vi "Line Pokayoke.vi"(8 "error in (no error)":errorcluster, 11 "Ref In":T6={"MS SQL Connection"=refnum, "UDL File"=path "", "Time"="", "DCODE"="", "WIP+1"=0, "MC No?"=0, "POKAYOKE?"=FALSE, "Expected Result"="", "Result [Status]"="", "Clock"=0.0, "RFID"="", "WIP Queue"=refnum, "TS Parameter"={"ProfitCenterCode"="", "LineCode"="", "WorkOrderNumber"="", "Model"="", "Model_with_Prefix"="", "VendorCode"="", "SetParameterDateCode"="", "PokaYoke"=0, "Target"=1, "Live_DateCode"="", "CustomerPartNumber"="", "Hand"="", "sBarcode"=FALSE, "FCA"=0, "Ent_Stamp"=timestamp(0 s since 1904-01-01), "STS_CD"=0.0}, "Data_Queue"=[], "RFID Serial No."=""} {"TS Parameter"."FCA" format="%01d"; "TS Parameter"."Target" min=1 max=100000; "TS Parameter"."PokaYoke" min=0 max=1}) -> (0 "error out":errorcluster)   [LabVIEW 2020]
uses:
  Controls/TD SQL.ctl
  <vilib>/addons/database/Connection.llb/Conn ObjectReference.ctl
  Controls/WIP_State.ctl
  Controls/TS_Parameter.ctl
  Controls/Line_PKYK.ctl
  Controls/PARA_CONTROL_STR.ctl
  Controls/PKYK_MCODE.ctl
  Controls/PKYK_DATE.ctl
  Controls/PKYK_Result.ctl
  <vilib>/Utility/miscctls.llb/LVPointTypeDef.ctl
  <vilib>/addons/database/Connection.llb/Conn Execute.vi
  <vilib>/addons/database/Recordset.llb/Rec Fetch Recordset Data (R).vi
  <vilib>/addons/database/NI_Database_API.lvlib
panel:
  in  "Hide":bool
  in  "OperationCode":T1 caption="Machine Code" items=["OP00", "OP10A", "OP10B", "OP20A", "OP20B", "OP30A", "OP30B", "OP30C", "OP40A", "OP40B", "OP50A", "OP50B", "OP60", "OP70", "OP80"]
  in  "MachineCode":T1 caption="Machine Code" items=["MCIG", "MCPC", "MCSA", "MCCA", "MCAC", "MCLA", "MCCM", "MCSC", "MCPA", "MCLP", "MCHP", "MCBC", "MCFA", "MCSR", "MCFV"]
  in  "PokaYokeNumber":string caption="PokaYoke Number"
  in  "Barcode":string
  in  "Part Number":string(combo)
  in  "PokaYoke Number":u16(ring) caption="PokaYokeNumber" items=["<New PokaYoke>", "00001", "00002", "00003", "00004", "00005", "00006", "00007", "00008", "00009", "00010", "00011", "00012", "00013", "00014", "00015", "00016"]
  in  "ExpiryDate":timestamp caption="Expiry Date" format="%<%d-%m-%Y>T"
  in  "Expected Result":T2
  in  "Description":string
  in  "Active Status":bool caption="IsActive"
  out "Date:":string
  out "Time:":string
  in  "Final Table":i32(listbox)
  in  "Refresh":bool
  in  "Print":bool
  in  "Exit":bool
  in  "Del":bool
  in  "change":bool
  in  "add":bool
  in  "PokaYoke Parameter":T3 {"MachineCode" items=["MCIG", "MCPC", "MCSA", "MCCA", "MCAC", "MCLA", "MCCM", "MCSC", "MCPA", "MCLP", "MCHP", "MCBC", "MCFA", "MCSR", "MCFV"]; "ExpiryDate" format="%<%I:%M:%S%3u %p\n%d-%m-%Y>T"; "EntDt" format="%<%I:%M:%S%3u %p\n%d-%m-%Y>T"; "UpdDt" format="%<%I:%M:%S%3u %p\n%d-%m-%Y>T"}
  # "Line Pokayoke"
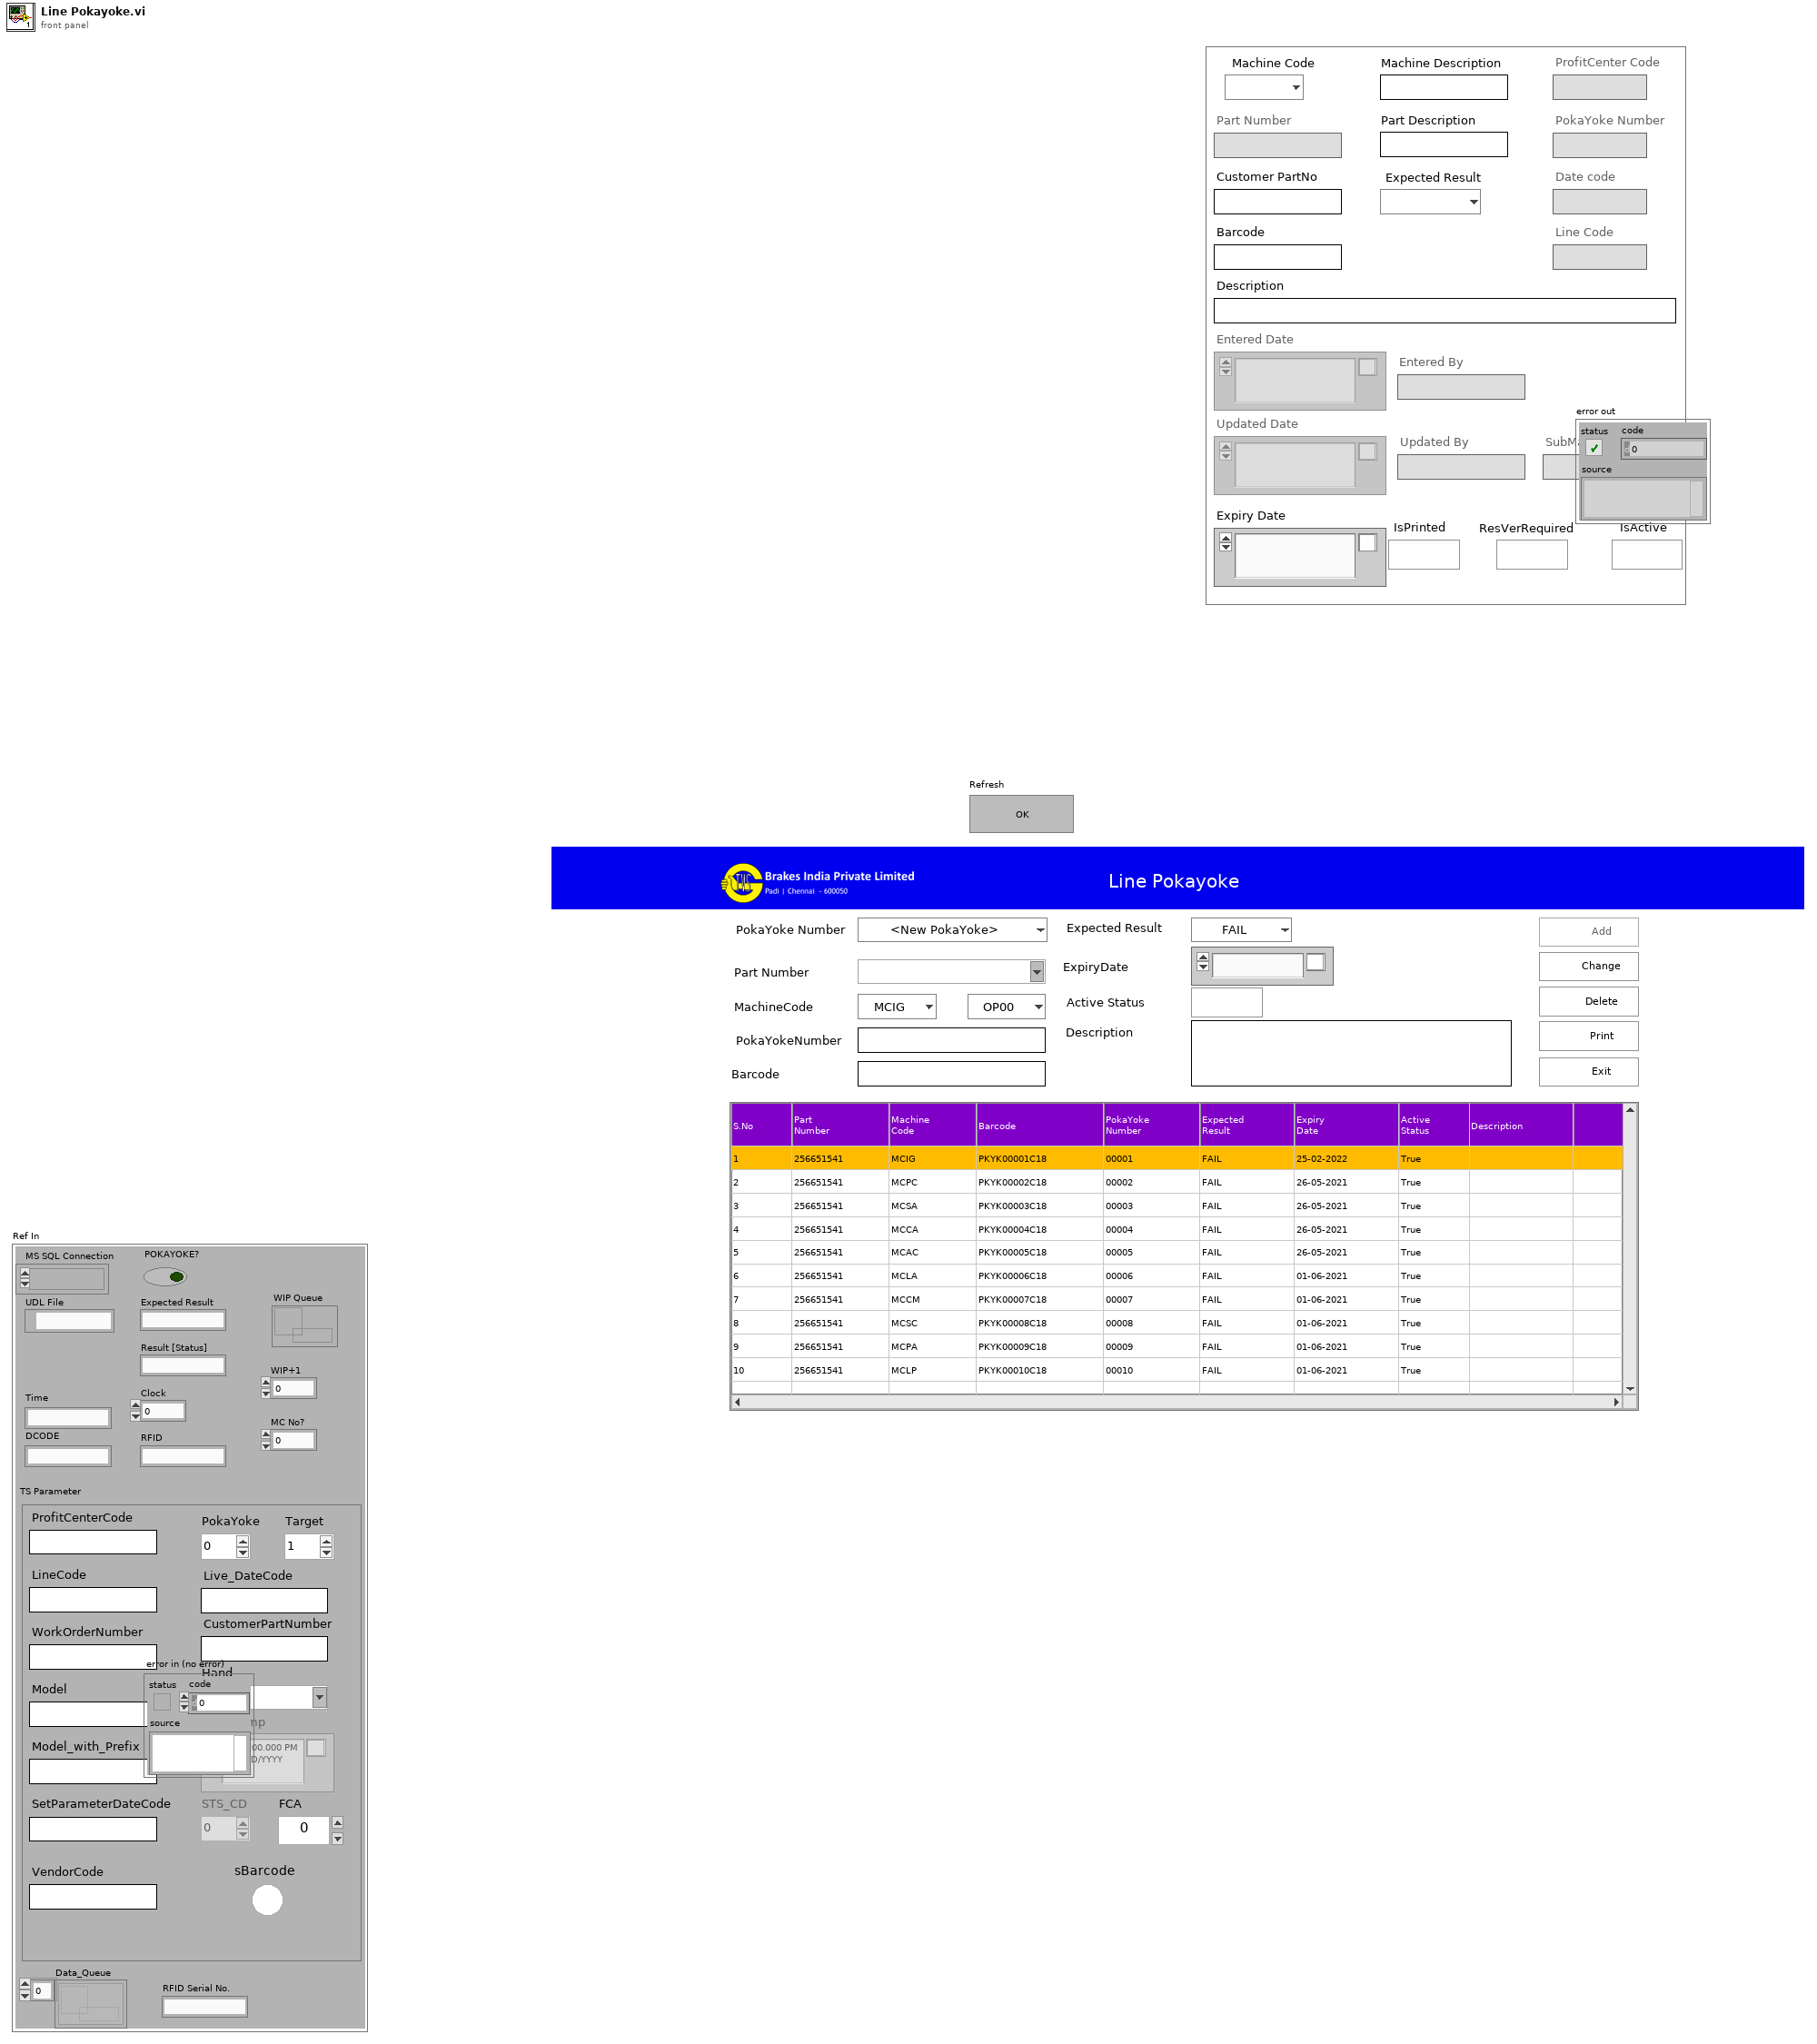
[diagram p1: front panel]
types:
  T1 = typedef "PKYK_MCODE.ctl" = u16
  T2 = typedef "PKYK_Result.ctl" = enum16{"FAIL", "PASS"}
  T3 = typedef "Line_PKYK.ctl" = cluster{"ProfitCenterCode":string, "LineCode":string, "Datecode":string, "PartNumber":T4, "PartDescription":T4, "CustPartNo":T4, "MachineCode":T1, "MachineDescription":T4, "PokaYokeNumber":string, "Description":string, "ExpiryDate":T5, "Barcode":T4, "IsPrinted":bool, "IsActive":bool, "EntBy":T4, "EntDt":T5, "UpdBy":T4, "UpdDt":T5, "ExpResult":T2, "ResVerRequired":bool, "SubMachineCode":T4}
  T4 = typedef "PARA_CONTROL_STR.ctl" = string
  T5 = typedef "PKYK_DATE.ctl" = timestamp
  T6 = typedef "TD SQL.ctl" = cluster{"MS SQL Connection":T7, "UDL File":path, "Time":string, "DCODE":string, "WIP+1":i64, "MC No?":i32, "POKAYOKE?":bool, "Expected Result":string, "Result [Status]":string, "Clock":dbl, "RFID":string, "WIP Queue":refnum<queue>, "TS Parameter":T8, "Data_Queue":refnum<queue>[], "RFID Serial No.":string}
  T7 = typedef "NI_Database_API.lvlib/Conn ObjectReference.ctl" = refnum<k1>
  T8 = typedef "TS_Parameter.ctl" = cluster{"ProfitCenterCode":string, "LineCode":string, "WorkOrderNumber":string, "Model":string, "Model_with_Prefix":string, "VendorCode":string, "SetParameterDateCode":string, "PokaYoke":i32, "Target":i32, "Live_DateCode":string, "CustomerPartNumber":string, "Hand":string, "sBarcode":bool, "FCA":i32, "Ent_Stamp":timestamp, "STS_CD":dbl}
  T9 = typedef "LVPointTypeDef.ctl" = cluster{"Horizontal":i16, "Vertical":i16}
  T10 = enum8{"Enabled", "Disabled", "Disabled and Grayed Out"}
  T11 = typedef "LVDateTimeRec.ctl" = cluster{"fractional second":dbl, "second":i32, "minute":i32, "hour":i32, "day of month":i32, "month":i32, "year":i32, "day of week":i32, "day of year":i32, "DST":i32}
  T12 = cluster{"s.nO":i32, "PartNumber":string, "MachineCode":string, "Barcode":string, "PokaYokeNumber":string, "ExpResult":string, "ExpiryDate":timestamp, "IsActive":bool, "Description":string}
  T13 = typedef "NI_Database_API.lvlib/Rec ObjectReference.ctl" = refnum<k1>
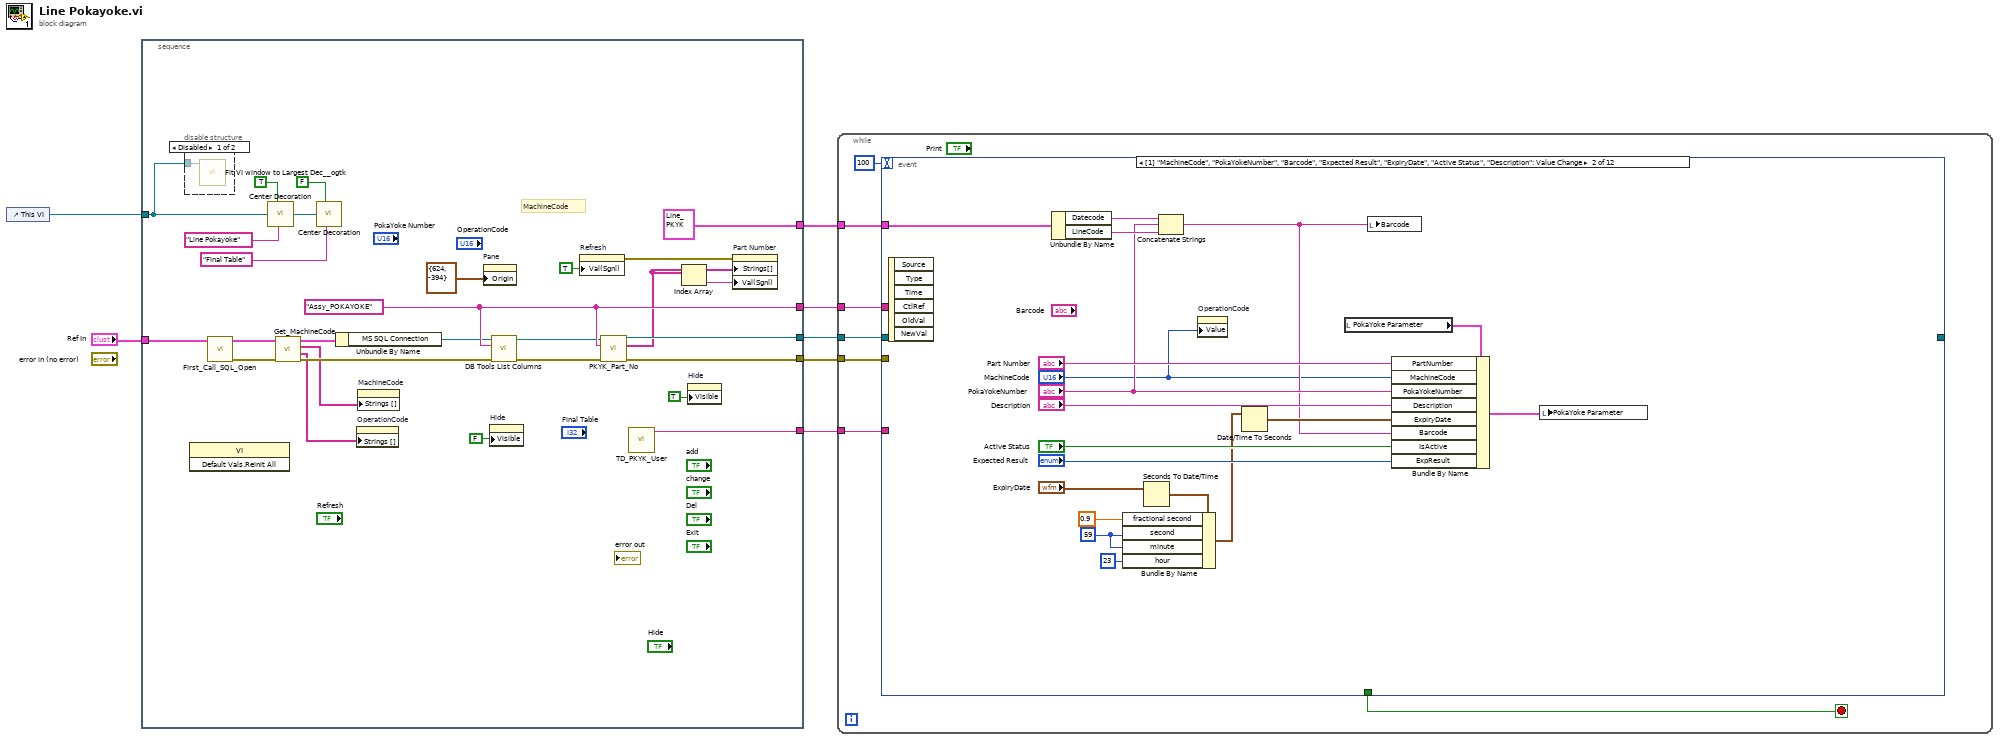
[diagram p0: block diagram]
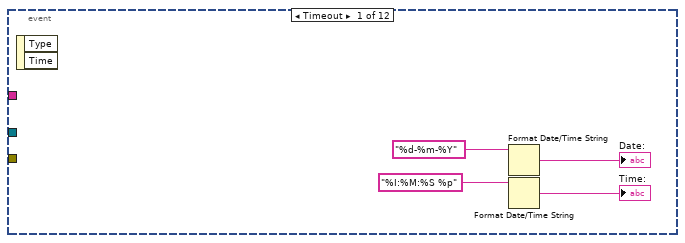
[diagram p2: hidden frame]
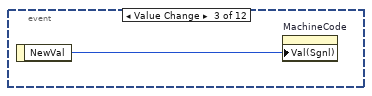
[diagram p3: hidden frame]
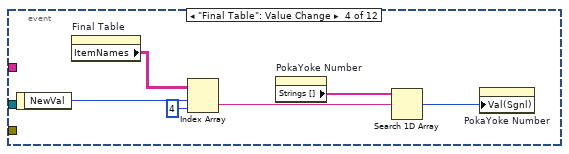
[diagram p4: hidden frame]
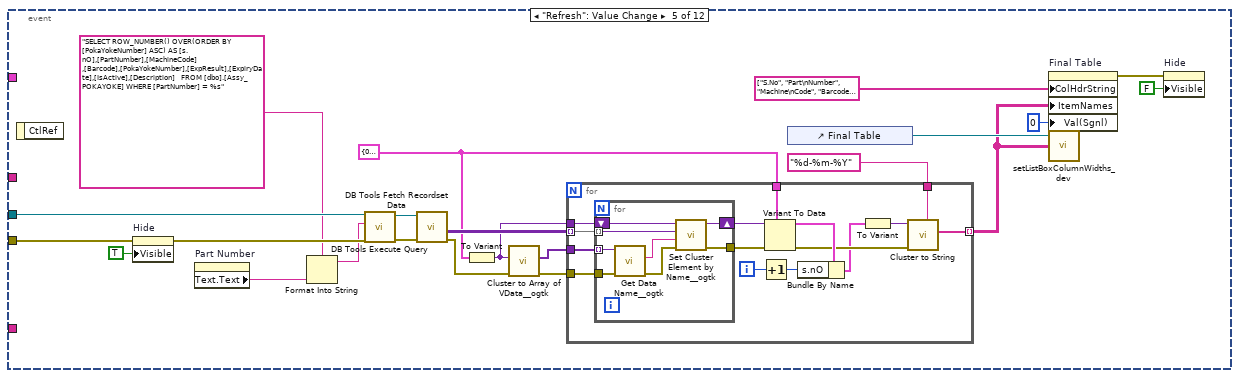
[diagram p5: hidden frame]
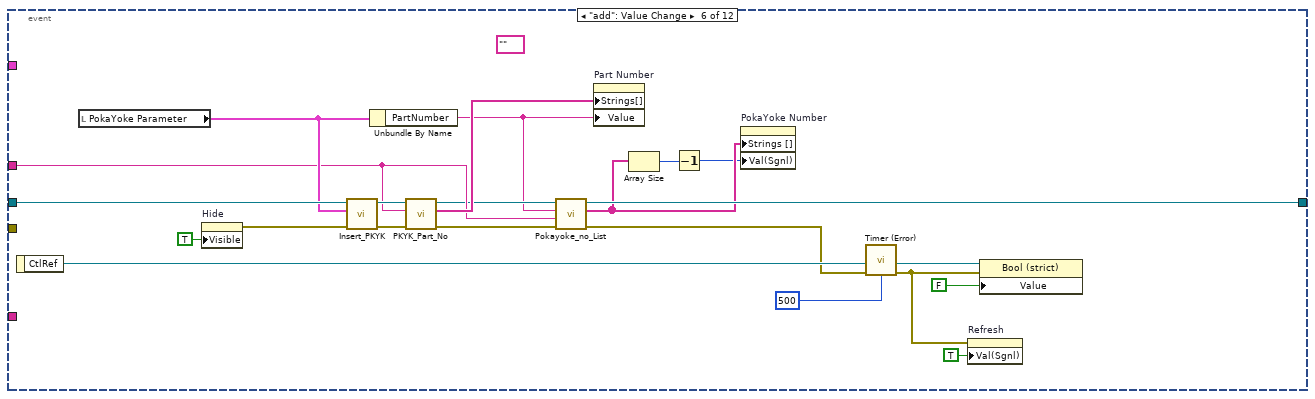
[diagram p6: hidden frame]
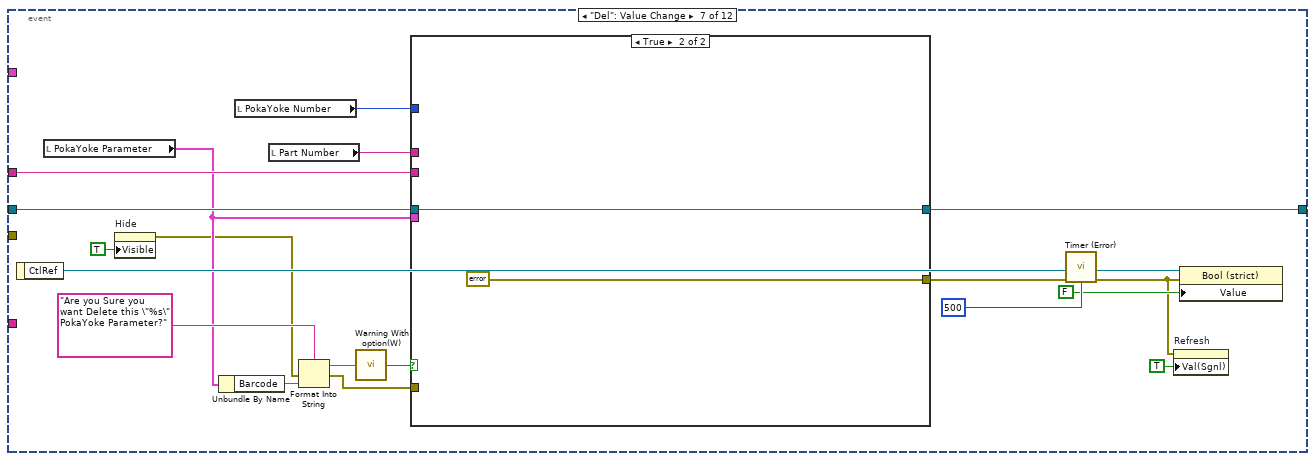
[diagram p7: hidden frame]
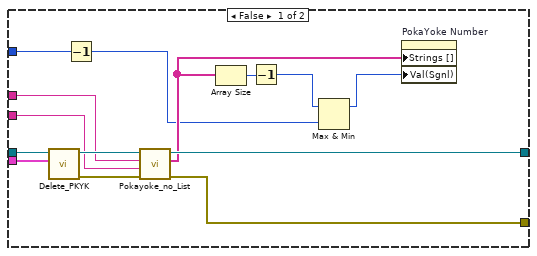
[diagram p8: hidden frame]
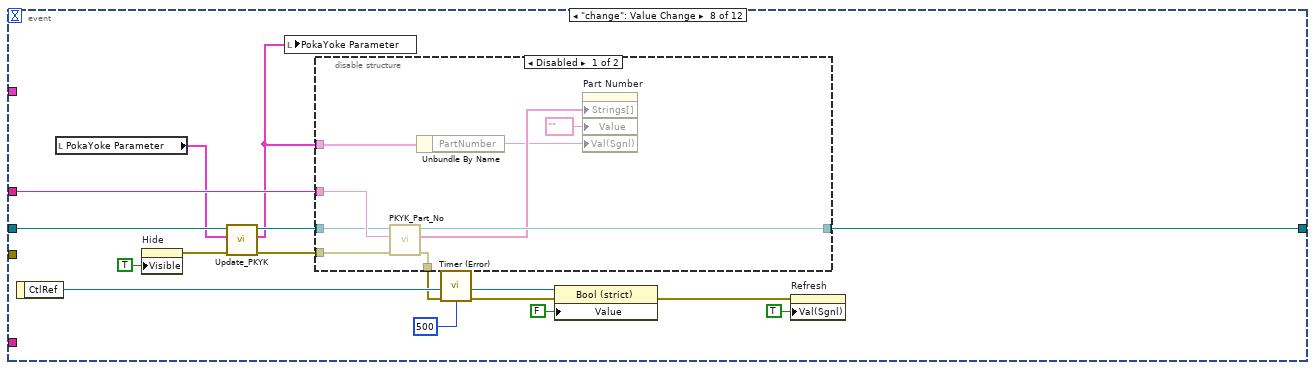
[diagram p9: hidden frame]
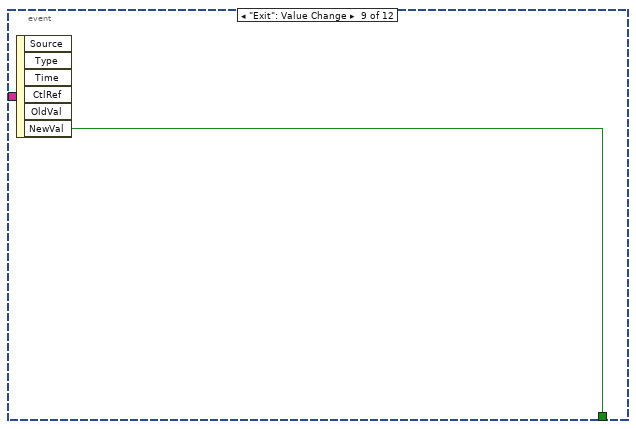
[diagram p11: hidden frame]
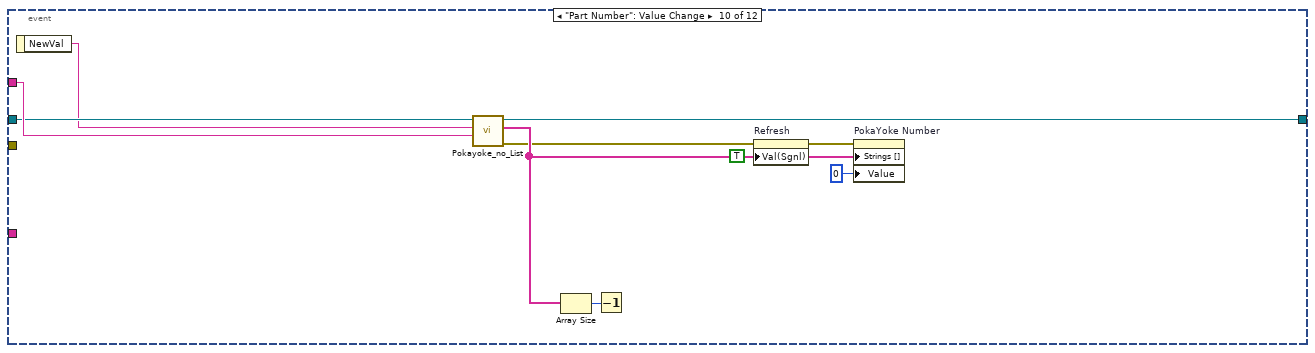
[diagram p12: hidden frame]
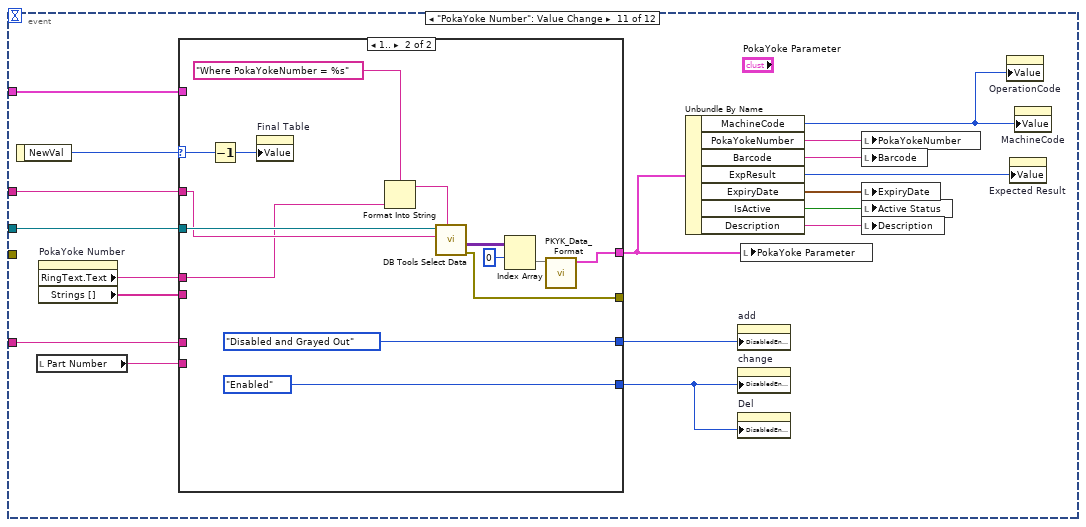
[diagram p13: hidden frame]
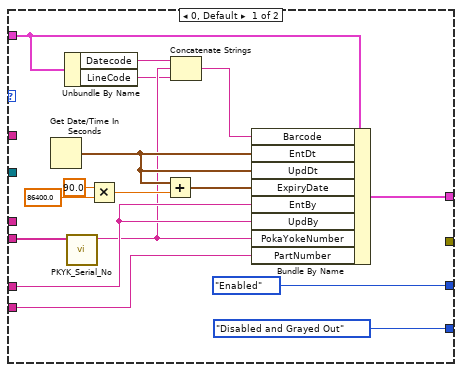
[diagram p14: hidden frame]
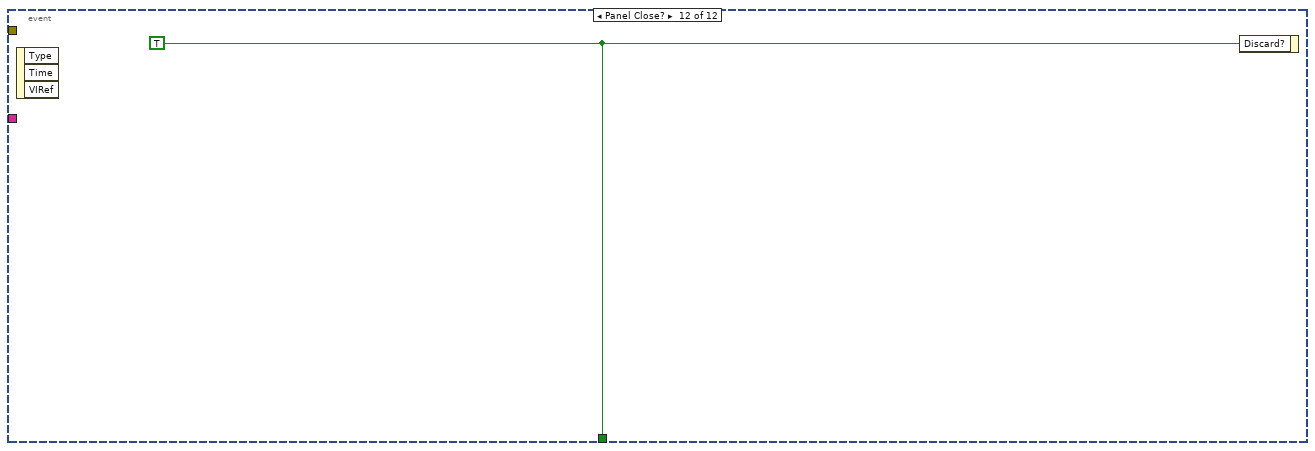
[diagram p15: hidden frame]
diagram:
  n1 = control-ref of="This VI"() -> (w1:refnum<vi>)
  n2 = stacked-sequence {
    tunnel: "Ref In" -> [w16]
    tunnel: [w34] -> w6
    tunnel: [w33] -> w5
    tunnel: [w32] -> w4
    tunnel: [T3 {"ProfitCenterCode"="0064", "LineCode"="C10", "Datecode"="PKYK", "PartNumber"="", "PartDescription"="", "CustPartNo"="", "MachineCode"=0, "MachineDescription"="", "PokaYokeNumber"="00008", "Description"="", "ExpiryDate"=timestamp(0 s since 1904-01-01), "Barcode"="PKYK00008C10", "IsPrinted"=TRUE, "IsActive"=TRUE, "EntBy"="ADMIN", "EntDt"=timestamp(0 s since 1904-01-01), "UpdBy"="ADMIN", "UpdDt"=timestamp(0 s since 1904-01-01), "ExpResult"=enum."FAIL", "ResVerRequired"=TRUE, "SubMachineCode"=""} ("Machine Code")] -> w3
    tunnel: [w26] -> w2
    tunnel: w1 -> [w13]
    frame #0 {
      w33 = "Assy_POKAYOKE" ("table")
      # "MachineCode"
      n3 = disable-structure shown="Disabled" {
        disable-tunnel: w13 -> [w36 _]
        frame Disabled {
          n4 = call <userlib>:"Fit VI window to Largest Dec__ogtk.vi"("VI Ref (calling VI)"=w36) -> ()  [unwired: 5 in, 2 out]
        }
        frame Enabled {
        }
      }
      n5 = invoke class="VI" method="Default Vals.Reinit All"() -> ()  [unwired: 3 in, 3 out]
      n6 = call "First_Call_SQL_Open.vi"("Ref In"=w16) -> ("error out"=w14:errorcluster, "Ref Out"=w15:T6)  [unwired: 9 in]
      n7 = call "Center Decoration.vi"("Decoration?"=TRUE, "VI in"=w13, "Object Name"="Line Pokayoke") -> ("VI out"=w10:refnum<vi>)  [unwired: 6 in]
      n8 = call "Get_MachineCode.vi"("error in (no error)"=w14, "Ref In"=w15) -> ("error out"=w19:errorcluster, "OperationCode"=w17:string[], "Machine Codes"=w18:string[], "Ref Out"=w20:T6)  [unwired: 6 in]
      n9 = call "Center Decoration.vi"("Decoration?"=FALSE, "VI in"=w10, "Object Name"="Final Table") -> ()  [unwired: 6 in, 1 out]
      n10 = Unbundle By Name(w20) -> ("MS SQL Connection"=w28:T7)
      n11 = property on="OperationCode" class="Ring (strict)"("Strings []"=w17) -> ()  [unwired: 2 in, 2 out]
      n12 = property on="MachineCode" class="Ring (strict)"("Strings []"=w18) -> ()  [unwired: 2 in, 2 out]
      n13 = property on="Pane" class="Pane"("Origin"=T9 {"Horizontal"=624, "Vertical"=-394}) -> ()  [unwired: 2 in, 2 out]
      n14 = property on="Hide" class="Bool"("Visible"=FALSE) -> ()  [unwired: 2 in, 2 out]
      n15 = call <vilib>:"DB Tools List Columns.vi"("error in (no error)"=w19, "table"=w33, "connection reference"=w28) -> ("error out"=w35:errorcluster, "connection reference out"=w27:T7)  [unwired: 1 in, 2 out]
      n16 = property on="Refresh" class="Bool (strict)"("Val(Sgnl)"=TRUE ("Value (Signaling)")) -> (error out=w24:errorcluster)  [unwired: 2 in, 1 out]
      n17 = call "PKYK_Part_No.vi"("error in (no error)"=w35, "table"=w33, "Refnum in"=w27) -> ("error out"=w26:errorcluster, "PKYK Part Number"=w31:string[], "Refnum out"=w34:T7)  [unwired: 6 in]
      n18 = call "TD_PKYK_User.vi"() -> ("User"=w32:string)  [unwired: 11 in]
      n19 = Index Array(array=w31) -> (element=w30:string)  [unwired: 1 in]
      n20 = property on="Hide" class="Bool"("Visible"=TRUE) -> ()  [unwired: 2 in, 2 out]
      n21 = property on="Part Number" class="CmbBox"(error in=w24, "Strings[]"=w31, "Val(Sgnl)"=w30) -> ()  [unwired: 1 in, 2 out]
    }
  }
  n22 = while {
    tunnel: w6 -> [w42]
    tunnel: w5 -> [w41]
    tunnel: w4 -> [w40]
    tunnel: w3 -> [w39]
    tunnel: w2 -> [w38]
    stop <- w43 stop-if-true
    n23 = event shown="[1] \"MachineCode\", \"PokaYokeNumber\", \"Barcode\", \"Expected Result\", \"ExpiryDate\", \"Active Status\", \"Description\": Value Change" {
      selector: _ -> [_ _ _ _ _ _ _ _ _ _ _ _]
      dyn-events: _ -> [_ _ _ _ _ _ _ _ _ _ _ _]
      timeout: 100 -> [_ _ _ _ _ _ _ _ _ _ _ _]
      tunnel: [_ _ _ _ _ _ _ _ w201 _ _ w260] -> w43
      tunnel: w42 -> [_ _ _ _ w95 w139 w158 w190 _ w210 w228 _]
      tunnel: w41 -> [_ _ _ _ _ w127 w155 w185 _ w211 w227 _]
      tunnel: w40 -> [_ _ _ _ _ _ _ _ _ _ w225 _]
      tunnel: w39 -> [_ w51 _ _ _ _ _ _ _ _ w224 _]
      tunnel: [_ _ _ _ _ w124 w154 w182 _ w206 _ _] -> _
      tunnel: w38 -> [_ _ _ _ w85 _ _ _ _ _ _ _]
      event Timeout {
        n24 = event-data() -> ()  [unwired: 1 in, 2 out]
        n25 = Format Date/Time String(time format string (%c)="%d-%m-%Y") -> (date/time string=→"Date:":string)  [unwired: 2 in]
        n26 = Format Date/Time String(time format string (%c)="%I:%M:%S %p") -> (date/time string=→"Time:":string)  [unwired: 2 in]
      }
      event "PokaYokeNumber", "Barcode", "ExpiryDate", "Active Status", "Description": Value Change {
        w55 = 59 ("second")
        n27 = event-data() -> ()  [unwired: 1 in, 6 out]
        n28 = Unbundle By Name(w51) -> ("Datecode"=w53:string, "LineCode"=w52:string)
        n29 = Seconds To Date/Time(time stamp (now)="ExpiryDate") -> (date time rec=w59:T11)  [unwired: 1 in]
        n30 = Bundle By Name(cluster=w59, "fractional second"=0.9, "second"=w55, "minute"=w55, "hour"=23) -> (w57:T11)
        n31 = Concatenate Strings(w53, "PokaYokeNumber", w52) -> (w49:string)
        n32 = property on="OperationCode" class="Ring (strict)"("Value"="MachineCode") -> ()  [unwired: 2 in, 2 out]
        n33 = Date/Time To Seconds(2:w57) -> (0:w58:timestamp)  [unwired: 1 in]
        n34 = local read "PokaYoke Parameter"() -> (w66:T3)
        n35 = local write "Barcode"(w49) -> ()
        n36 = Bundle By Name(cluster=w66, "PartNumber"="Part Number", "MachineCode"="MachineCode", "PokaYokeNumber"="PokaYokeNumber", "Description"="Description", "ExpiryDate"=w58, "Barcode"=w49, "IsActive"="Active Status", "ExpResult"="Expected Result") -> (w65:T3)
        n37 = local write "PokaYoke Parameter"(w65) -> ()
      }
      event Value Change {
        n38 = event-data() -> ("NewVal"=w67:T1)  [unwired: 1 in]
        n39 = property on="MachineCode" class="Ring (strict)"("Val(Sgnl)"=w67) -> ()  [unwired: 2 in, 2 out]
      }
      event "Final Table": Value Change {
        n40 = event-data() -> ("NewVal"=w72:i32)  [unwired: 1 in]
        n41 = property on="Final Table" class="MCListbox (strict)"() -> ("ItemNames"=w73:string[][])  [unwired: 2 in, 2 out]
        n42 = Index Array(array=w73, index (row)=w72, index (col)=4 ("disabled index (col)")) -> (element=w69:string)
        n43 = property on="PokaYoke Number" class="Ring (strict)"() -> ("Strings []"=w70:string[])  [unwired: 2 in, 2 out]
        n44 = Search 1D Array(1D array=w70, element=w69) -> (index of element=w68:i32)  [unwired: 1 in]
        n45 = property on="PokaYoke Number" class="Ring (strict)"("Val(Sgnl)"=w68) -> ()  [unwired: 2 in, 2 out]
      }
      event "Refresh": Value Change {
        w88 = T12 {"s.nO"=0, "PartNumber"="", "MachineCode"="", "Barcode"="", "PokaYokeNumber"="", "ExpResult"="", "ExpiryDate"=timestamp(0 s since 1904-01-01), "IsActive"=FALSE, "Description"=""} ("Cluster")
        n46 = event-data() -> ()  [unwired: 1 in, 1 out]
        n47 = property on="Hide" class="Bool"(error in=w85, "Visible"=TRUE) -> (error out=w84:errorcluster)  [unwired: 1 in, 1 out]
        n48 = property on="Part Number" class="CmbBox"() -> ("Text.Text"=w75:string)  [unwired: 2 in, 2 out]
        n49 = Format Into String(format string="SELECT ROW_NUMBER() OVER(ORDER BY [PokaYokeNumber] ASC) AS [s.nO],[PartNumber],[MachineCode] ,[Barcode],[PokaYokeNumber],[ExpResult],[ExpiryDate],[IsActive],[Description]   FROM [dbo].[Assy_POKAYOKE] WHERE [PartNumber] = %s", w75) -> (resulting string=w76:string)  [unwired: 2 in, 1 out]
        n50 = call-poly <vilib>:"DB Tools Execute Query.vi"("error in (no error)"=w84, "SQL query"=w76, "connection reference"=w95) -> ("error out"=w80:errorcluster, "recordset reference"=w81:T13)  [unwired: 5 in]
        n51 = call-poly <vilib>:"DB Tools Fetch Recordset Data.vi"("error in (no error)"=w80, "recordset reference"=w81) -> ("error out"=w79:errorcluster, "recordset data"=w92:variant[][])  [unwired: 3 in, 1 out]
        n52 = To Variant(anything=w88) -> (Variant=w90:variant)
        n53 = call <userlib>:"Cluster to Array of VData__ogtk.vi"("error in (no error)"=w79, "Cluster"=w90) -> ("error out"=w78:errorcluster, "Array of VData"=w91:variant[])  [unwired: 8 in]
        n54 = for {
          tunnel: w92 -> [w110] mode=indexing
          tunnel: w90 -> [w108]
          tunnel: w91 -> [w109]
          tunnel: [w106] -> w89 mode=indexing
          tunnel: w88 -> [w102]
          tunnel: "%d-%m-%Y" ("time format string (%c)") -> [w97]
          tunnel: w78 -> [w96]
          i -> [w99]
          n55 = for {
            tunnel: w110 -> [w117] mode=indexing
            tunnel: w109 -> [w116] mode=indexing
            shift-right: [w114] -> w107
            shift-left: w108 -> [w118]
            tunnel: [w113] -> w105
            tunnel: w96 -> [w111]
            n56 = call <userlib>:"Get Data Name__ogtk.vi"("error in (no error)"=w111, "Data"=w116) -> ("error out"=w115:errorcluster, "Data Name"=w112:string)  [unwired: 7 in, 1 out]
            n57 = call <userlib>:"Set Cluster Element by Name__ogtk.vi"("error in (no error)"=w115, "Element Name (\"\": New Element Data Name)"=w112, "New Element Value"=w117, "Cluster"=w118) -> ("error out"=w113:errorcluster, "VCluster out"=w114:variant)  [unwired: 5 in, 1 out]
          }
          n58 = Increment(x=w99) -> (x+1=w98:i32)
          n59 = Variant To Data(error in=w105, type=w102, Variant=w107) -> (data=w104:T12, error out=w103:errorcluster)
          n60 = Bundle By Name(cluster=w104, "s.nO"=w98) -> (w100:T12)
          n61 = To Variant(anything=w100) -> (Variant=w101:variant)
          n62 = call <userlib>:"Cluster to String.vi"("Time Format String"=w97, "error in (no error)"=w103, "Variant In"=w101) -> ("Format String Array"=w106:string[])  [unwired: 5 in, 3 out]
        }
        n63 = control-ref of="Final Table"() -> (w94:refnum<vi>)
        n64 = property on="Final Table" class="MCListbox (strict)"("ColHdrString"=string[] ["S.No", "Part\nNumber", "Machine\nCode", "Barcode", "PokaYoke\nNumber", "Expected \nResult", "Expiry\nDate", "Active\nStatus", "Description"] ("Item Names"), "ItemNames"=w89, "Val(Sgnl)"=0 ("Value (Signaling)")) -> (error out=w82:errorcluster)  [unwired: 2 in, 1 out]
        n65 = call "setListBoxColumnWidths_dev.vi"("table data"=w89, "MCListbox Refnum"=w94) -> ()  [unwired: 1 in]
        n66 = property on="Hide" class="Bool"(error in=w82, "Visible"=FALSE) -> ()  [unwired: 1 in, 2 out]
      }
      event "add": Value Change {
        (unwired) "" ("Part Number")
        n67 = event-data() -> ("CtlRef"=w138:refnum<vi>)  [unwired: 1 in]
        n68 = local read "PokaYoke Parameter"() -> (w132:T3)
        n69 = property on="Hide" class="Bool"("Visible"=TRUE) -> (error out=w128:errorcluster)  [unwired: 2 in, 1 out]
        n70 = call "Insert_PKYK.vi"("error in (no error)"=w128, "PokaYoke Parameter"=w132, "Refnum in"=w139) -> ("error out"=w135:errorcluster, "Refnum out"=w134:T7)  [unwired: 7 in]
        n71 = Unbundle By Name(w132) -> ("PartNumber"=w122:T4)
        n72 = call "PKYK_Part_No.vi"("error in (no error)"=w135, "table"=w127, "Refnum in"=w134) -> ("error out"=w126:errorcluster, "PKYK Part Number"=w133:string[], "Refnum out"=w125:T7)  [unwired: 6 in]
        n73 = call "Pokayoke_no_List.vi"("error in (no error)"=w126, "Table Name"=w127, "Part Number"=w122, "Refnum in"=w125) -> ("error out"=w123:errorcluster, "Pokayoke List"=w121:string[], "Refnum out"=w124:T7)  [unwired: 5 in]
        n74 = property on="Part Number" class="CmbBox"("Strings[]"=w133, "Value"=w122) -> ()  [unwired: 2 in, 2 out]
        n75 = Array Size(array=w121) -> (size(s)=w120:i32)
        n76 = Decrement(x=w120) -> (x-1=w119:i32)
        n77 = property on="PokaYoke Number" class="Ring (strict)"("Strings []"=w121, "Val(Sgnl)"=w119) -> ()  [unwired: 2 in, 2 out]
        n78 = call <userlib>:"Timer (Error).vi"("error in (no error)"=w123, "milliseconds to wait"=u32 500) -> ("error out"=w130:errorcluster)  [unwired: 13 in]
        n79 = property on="Refresh" class="Bool (strict)"(error in=w130, "Val(Sgnl)"=TRUE ("Value (Signaling)")) -> ()  [unwired: 1 in, 2 out]
        n80 = property class="Bool (strict)"(reference=w138, error in=w130, "Value"=FALSE) -> ()  [unwired: 2 out]
      }
      event "Del": Value Change {
        n81 = event-data() -> ("CtlRef"=w157:refnum<vi>)  [unwired: 1 in]
        n82 = local read "PokaYoke Parameter"() -> (w151:T3)
        n83 = property on="Hide" class="Bool"("Visible"=TRUE) -> (error out=w140:errorcluster)  [unwired: 2 in, 1 out]
        n84 = Unbundle By Name(w151) -> ("Barcode"=w150:T4)
        n85 = local read "PokaYoke Number"() -> (w147:u16)
        n86 = local read "Part Number"() -> (w146:string)
        n87 = Format Into String(format string="Are you Sure you want Delete this \"%s\" PokaYoke Parameter?" ("Warning in"), error in=w140, w150) -> (resulting string=w149:string, error out=w145:errorcluster)  [unwired: 1 in]
        n88 = call <userlib>:"Warning With option(W).vi"("Warning in"=w149) -> ("Cancel ?"=w148:bool)  [unwired: 13 in, 1 out]
        n89 = case shown="True" w148 {
          tunnel: w158 -> [w172 w174]
          tunnel: w155 -> [w169 _]
          tunnel: [w166 w174] -> w154
          tunnel: [w167 errorcluster {"status"=FALSE, "code"=0, "source"=""} ("error out")] -> w153
          tunnel: w151 -> [w171 _]
          tunnel: w147 -> [w162 _]
          tunnel: w146 -> [w165 _]
          tunnel: w145 -> [_ _]
          frame False {
            n90 = call "Delete_PKYK.vi"("PokaYoke In"=w171, "Refnum in"=w172) -> ("error out"=w168:errorcluster, "Refnum out"=w170:T7)  [unwired: 8 in]
            n91 = Decrement(x=w162) -> (x-1=w160:u16)
            n92 = call "Pokayoke_no_List.vi"("error in (no error)"=w168, "Table Name"=w169, "Part Number"=w165, "Refnum in"=w170) -> ("error out"=w167:errorcluster, "Pokayoke List"=w163:string[], "Refnum out"=w166:T7)  [unwired: 5 in]
            n93 = Array Size(array=w163) -> (size(s)=w164:i32)
            n94 = Decrement(x=w164) -> (x-1=w161:i32)
            n95 = Max & Min(x=w161, y=w160) -> (max(x,y)=w159:i32)  [unwired: 1 out]
            n96 = property on="PokaYoke Number" class="Ring (strict)"("Strings []"=w163, "Val(Sgnl)"=w159) -> ()  [unwired: 2 in, 2 out]
          }
          frame True {
          }
        }
        n97 = call <userlib>:"Timer (Error).vi"("error in (no error)"=w153, "milliseconds to wait"=u32 500) -> ("error out"=w142:errorcluster)  [unwired: 13 in]
        n98 = property on="Refresh" class="Bool (strict)"(error in=w142, "Val(Sgnl)"=TRUE ("Value (Signaling)")) -> ()  [unwired: 1 in, 2 out]
        n99 = property class="Bool (strict)"(reference=w157, error in=w142, "Value"=FALSE) -> ()  [unwired: 2 out]
      }
      event "change": Value Change {
        n100 = event-data() -> ("CtlRef"=w189:refnum<vi>)  [unwired: 1 in]
        n101 = local read "PokaYoke Parameter"() -> (w180:T3)
        n102 = property on="Hide" class="Bool"("Visible"=TRUE) -> (error out=w175:errorcluster)  [unwired: 2 in, 1 out]
        n103 = call "Update_PKYK.vi"("error in (no error)"=w175, "PokaYoke In"=w180, "Refnum in"=w190) -> ("error out"=w184:errorcluster, "PokaYoke Out"=w179:T3, "Refnum out"=w183:T7)  [unwired: 6 in]
        n104 = local write "PokaYoke Parameter"(w179) -> ()
        n105 = disable-structure shown="Disabled" {
          disable-tunnel: w185 -> [w198 _]
          disable-tunnel: w184 -> [w197 _]
          disable-tunnel: w183 -> [w196 w200]
          disable-tunnel: [w195 w200] -> w182
          disable-tunnel: [w194 _] -> w181
          disable-tunnel: w179 -> [w191 _]
          frame Disabled {
            n106 = call "PKYK_Part_No.vi"("error in (no error)"=w197, "table"=w198, "Refnum in"=w196) -> ("error out"=w194:errorcluster, "PKYK Part Number"=w193:string[], "Refnum out"=w195:T7)  [unwired: 6 in]
            n107 = Unbundle By Name(w191) -> ("PartNumber"=w192:T4)
            n108 = property on="Part Number" class="CmbBox"("Strings[]"=w193, "Value"="" ("Part Number"), "Val(Sgnl)"=w192) -> ()  [unwired: 2 in, 2 out]
          }
          frame Enabled {
          }
        }
        n109 = call <userlib>:"Timer (Error).vi"("error in (no error)"=w181, "milliseconds to wait"=u32 500) -> ("error out"=w186:errorcluster)  [unwired: 13 in]
        n110 = property class="Bool (strict)"(reference=w189, error in=w186, "Value"=FALSE) -> (error out=w177:errorcluster)  [unwired: 1 out]
        n111 = property on="Refresh" class="Bool (strict)"(error in=w177, "Val(Sgnl)"=TRUE ("Value (Signaling)")) -> ()  [unwired: 1 in, 2 out]
      }
      event "Exit": Value Change {
        n112 = event-data() -> ("NewVal"=w201:bool)  [unwired: 1 in, 5 out]
      }
      event "Part Number": Value Change {
        n113 = event-data() -> ("NewVal"=w209:string)  [unwired: 1 in]
        n114 = call "Pokayoke_no_List.vi"("Table Name"=w211, "Part Number"=w209, "Refnum in"=w210) -> ("error out"=w202:errorcluster, "Pokayoke List"=w207:string[], "Refnum out"=w206:T7)  [unwired: 6 in]
        n115 = Array Size(array=w207) -> (size(s)=w208:i32)
        n116 = Decrement(x=w208) -> ()  [unwired: 1 out]
        n117 = property on="Refresh" class="Bool (strict)"(error in=w202, "Val(Sgnl)"=TRUE ("Value (Signaling)")) -> (error out=w203:errorcluster)  [unwired: 1 in, 1 out]
        n118 = property on="PokaYoke Number" class="Ring (strict)"(error in=w203, "Strings []"=w207, "Value"=u16 0 ("Value (Signaling)")) -> ()  [unwired: 1 in, 2 out]
      }
      event "PokaYoke Number": Value Change {
        n119 = event-data() -> ("NewVal"=w229:u16)  [unwired: 1 in]
        n120 = local read "Part Number"() -> (w222:string)
        n121 = property on="PokaYoke Number" class="Ring (strict)"() -> ("RingText.Text"=w226:string, "Strings []"=w223:string[])  [unwired: 2 in, 2 out]
        n122 = case shown="1.." w229 {
          selector: w229 -> [_ w248]
          tunnel: w228 -> [_ w259]
          tunnel: w227 -> [_ w258]
          tunnel: w226 -> [_ w255]
          tunnel: [w245 w251] -> w219
          tunnel: w225 -> [w239 _]
          tunnel: w224 -> [w237 _]
          tunnel: w223 -> [w238 _]
          tunnel: w222 -> [w232 _]
          tunnel: [T10."Enabled" ("Disabled") T10."Disabled and Grayed Out" ("Disabled")] -> w221
          tunnel: [T10."Disabled and Grayed Out" ("Disabled") T10."Enabled" ("Disabled")] -> w220
          tunnel: [_ w246] -> _
          frame 0, Default {
            n123 = Get Date/Time In Seconds() -> (seconds since 1Jan1904=w242:timestamp)
            n124 = Unbundle By Name(w237) -> ("Datecode"=w236:string, "LineCode"=w234:string)
            n125 = call "PKYK_Serial_No.vi"("Strings []"=w238) -> ("Serial Number"=w235:string)  [unwired: 10 in]
            n126 = Multiply(x=90.0, y=86400.0) -> (x*y=w241:dbl)
            n127 = Add(x=w242, y=w241) -> (x+y=w240:timestamp)
            n128 = Concatenate Strings(w236, w235, w234) -> (w233:string)
            n129 = Bundle By Name(cluster=w237, "Barcode"=w233, "EntDt"=w242, "UpdDt"=w242, "ExpiryDate"=w240, "EntBy"=w239, "UpdBy"=w239, "PokaYokeNumber"=w235, "PartNumber"=w232) -> (w245:T3)
          }
          frame 1.. {
            n130 = Decrement(x=w248) -> (x-1=w247:u16)
            n131 = property on="Final Table" class="MCListbox (strict)"("Value"=w247) -> ()  [unwired: 2 in, 2 out]
            n132 = Format Into String(format string="Where PokaYokeNumber = %s" ("String"), w255) -> (resulting string=w256:string)  [unwired: 2 in, 1 out]
            n133 = call <vilib>:"DB Tools Select Data.vi"("condition"=w256, "table"=w258, "connection reference"=w259) -> ("error out"=w246:errorcluster, "data"=w254:variant[][])  [unwired: 3 in, 1 out]
            n134 = Index Array(array=w254, index (row)=0 ("disabled index (col)")) -> (element=w252:variant[])  [unwired: 1 in]
            n135 = call "PKYK_Data_Format.vi"("Pokayoke Data"=w252) -> ("Pokayoke Data Out"=w251:T3)  [unwired: 10 in]
          }
        }
        n136 = Unbundle By Name(w219) -> ("MachineCode"=w212:T1, "PokaYokeNumber"=w218:string, "Barcode"=w217:T4, "ExpResult"=w216:T2, "ExpiryDate"=w215:T5, "IsActive"=w214:bool, "Description"=w213:string)
        n137 = property on="add" class="Bool (strict)"("DisabledEnum"=w221) -> ()  [unwired: 2 in, 2 out]
        n138 = property on="change" class="Bool (strict)"("DisabledEnum"=w220) -> ()  [unwired: 2 in, 2 out]
        n139 = property on="Del" class="Bool (strict)"("DisabledEnum"=w220) -> ()  [unwired: 2 in, 2 out]
        n140 = local write "PokaYoke Parameter"(w219) -> ()
        n141 = local write "PokaYokeNumber"(w218) -> ()
        n142 = local write "Barcode"(w217) -> ()
        n143 = local write "ExpiryDate"(w215) -> ()
        n144 = local write "Active Status"(w214) -> ()
        n145 = local write "Description"(w213) -> ()
        n146 = property on="OperationCode" class="Ring (strict)"("Value"=w212) -> ()  [unwired: 2 in, 2 out]
        n147 = property on="Expected Result" class="Enum (strict)"("Value"=w216) -> ()  [unwired: 2 in, 2 out]
        n148 = property on="MachineCode" class="Ring (strict)"("Value"=w212) -> ()  [unwired: 2 in, 2 out]
      }
      event Panel Close? {
        w260 = TRUE ("Discard?")
        n149 = event-data() -> ()  [unwired: 1 in, 3 out]
        n150 = event-data("Discard?"=w260) -> ()  [unwired: 1 in, 1 out]
      }
    }
  }
